vi "Actor Core.vi"(8 "error in":errorcluster, 11 "Nested in":refnum<class "UI.lvclass">) -> (0 "error out":errorcluster, 3 "Actor out":refnum<class "Actor.lvclass">)   [LabVIEW 2020, in "UI.lvlib" / "UI.lvclass"]
doc: "(<B>Filename</B>: Actor Framework.lvlib:Actor.lvclass:Actor Core.vi)\n\nReceives messages to the actor, reacts to them, and initiates any error handling that may shut the actor down.\n\nDescendant classes may override this VI to append parallel tasks for the actor to complete while it handles messages. Overrides use the Call Parent Method node."
uses:
  UI.lvclass
  C:/Program Files (x86)/National Instruments/LabVIEW 2020/vi.lib/ActorFramework/Actor/Actor.lvclass
  <vilib>/ActorFramework/Actor/Actor.lvclass
  Turnos/Turnos.lvclass
  Paquetes/Paquetes.lvclass
  Dinero/Dinero.lvclass
  Contabilidad/Contabilidad.lvclass
  UI.lvclass/UI.ctl
  Turnos/Turnos.lvclass/Turnos.ctl
  Paquetes/Paquetes.lvclass/Paquetes.ctl
  Dinero/Dinero.lvclass/Dinero.ctl
  <vilib>/ActorFramework/Actor/Actor.lvclass/Actor.ctl
  <vilib>/ActorFramework/Message Enqueuer/Message Enqueuer.lvclass/Message Enqueuer.ctl
  UI Messages/New Credit and cambio to Dinero Msg/New Credit and cambio to Dinero Msg.lvclass/New Credit and cambio to Dinero Msg.ctl
  UI Messages/Verificar Credito Msg/Verificar Credito Msg.lvclass/Verificar Credito Msg.ctl
  UI Messages/UI Mensaje to Paquetes Msg/UI Mensaje to Paquetes Msg.lvclass/UI Mensaje to Paquetes Msg.ctl
  UI Messages/Servicio to contabilidad Msg/Servicio to contabilidad Msg.lvclass/Servicio to contabilidad Msg.ctl
  <vilib>/ActorFramework/Message Enqueuer/Init from Existing Queue.vi
  <vilib>/ActorFramework/Message Enqueuer/Enqueue.vi
  <vilib>/ActorFramework/Stop Msg/Stop Msg.lvclass
  C:/Program Files (x86)/National Instruments/LabVIEW 2020/vi.lib/ActorFramework/Message/Message.lvclass
  UI Messages/New Credit and cambio to Dinero Msg/New Credit and cambio to Dinero Msg.lvclass
  UI Messages/Verificar Credito Msg/Verificar Credito Msg.lvclass
  UI Messages/UI Mensaje to Paquetes Msg/UI Mensaje to Paquetes Msg.lvclass
  UI Messages/Servicio to contabilidad Msg/Servicio to contabilidad Msg.lvclass
  <vilib>/ActorFramework/Message Priority Queue/Priority Enqueue.vi
  <vilib>/ActorFramework/Message Enqueuer/Message Enqueuer.lvclass
  UI Messages/Table to Turnos Msg/Table to Turnos Msg.lvclass
panel:
  out "New Credit":i32
  out "SERIVICIO":string
  out "Cambio":i32
  out "Credito":i32
  in  "Contabilidad":bool
  in  "Stop Total":bool
  in  "Stop":bool
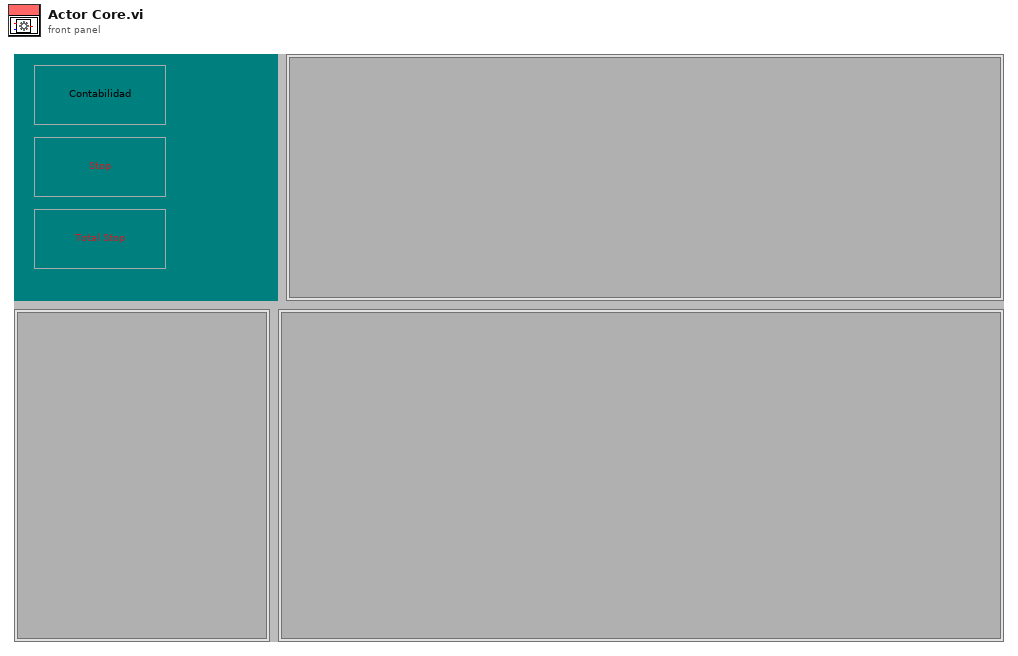
[diagram p1: front panel]
types:
  T1 = cluster{"Stop":refnum<user-event>, "Credito":refnum<user-event>, "Cambio":refnum<user-event>, "SERIVICIO":refnum<user-event>, "Mensaje":refnum<user-event>, "New Credit":refnum<user-event>, "Tabla estatus":refnum<user-event>}
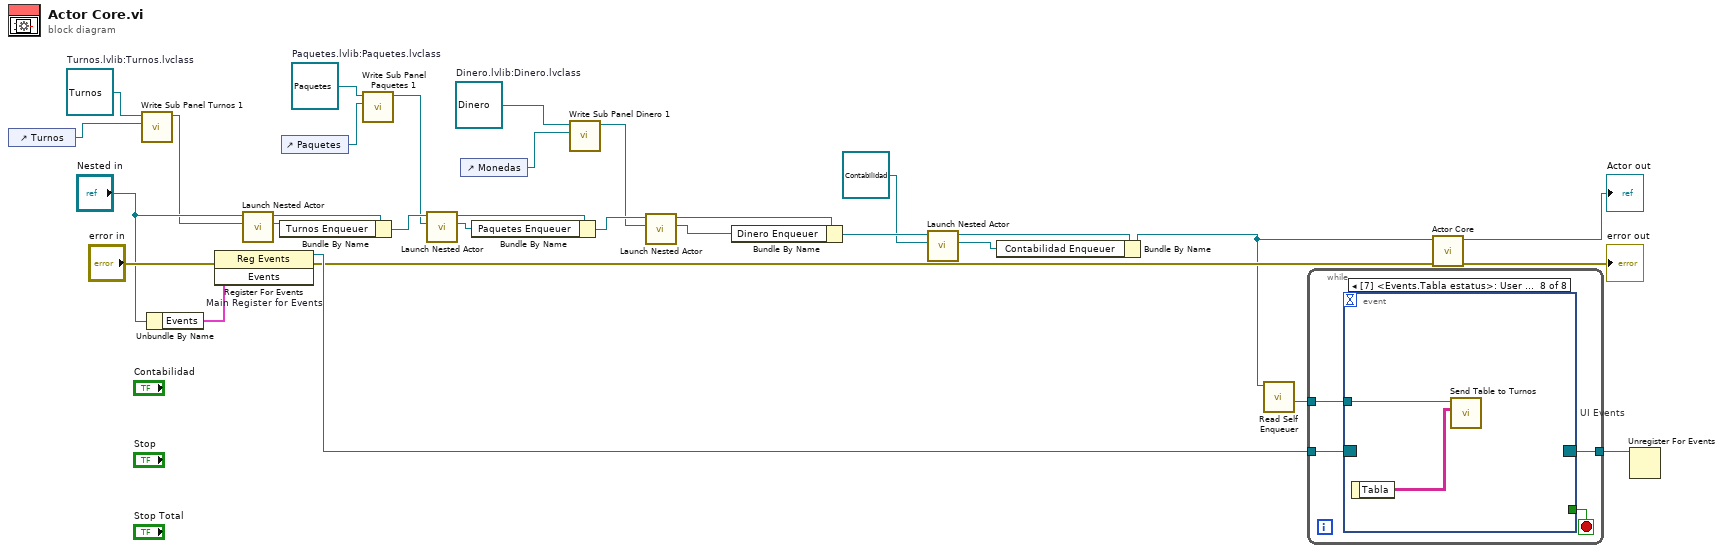
[diagram p0: block diagram]
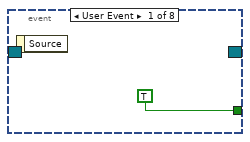
[diagram p2: hidden frame]
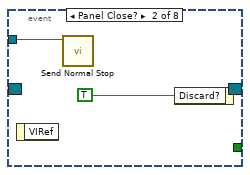
[diagram p3: hidden frame]
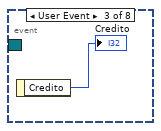
[diagram p4: hidden frame]
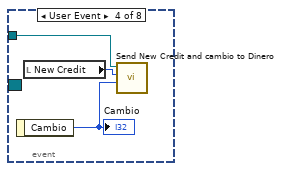
[diagram p5: hidden frame]
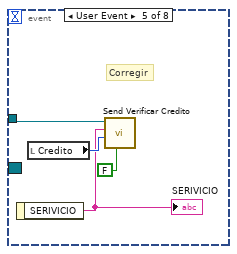
[diagram p6: hidden frame]
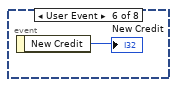
[diagram p7: hidden frame]
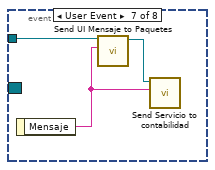
[diagram p8: hidden frame]
diagram:
  w10 = refnum<class "Dinero.lvclass"> refnum  # Dinero.lvlib:Dinero.lvclass
  w17 = refnum<class "Paquetes.lvclass"> refnum  # Paquetes.lvlib:Paquetes.lvclass
  w23 = refnum<class "Turnos.lvclass"> refnum  # Turnos.lvlib:Turnos.lvclass
  n1 = control-ref of="Turnos"() -> (w21:refnum<vi>)
  n2 = call "Write Sub Panel Turnos 1.vi"("Sub Panel Turnos"=w21, "Turnos in"=w23) -> ("Turnos out"=w20:refnum<class "Turnos.lvclass">)  [unwired: 8 in, 1 out]
  n3 = Unbundle By Name("Nested in") -> ("Events"=w28:T1)
  n4 = register-events "Main Register for Events"(error in="error in", w28) -> (reference out=w29:refnum<event-registration>, error out=w24:errorcluster)  [unwired: 1 in]
  n5 = call <vilib>:"Launch Nested Actor.vi"("Nested Actor"=w20, "Caller Actor in"="Nested in") -> ("Nested Actor's Enqueuer"=w18:refnum<class "Message Enqueuer.lvclass">, "Caller Actor out"=w19:refnum<class "UI.lvclass">)  [unwired: 7 in, 1 out]
  n6 = Bundle By Name(cluster=w19, "Turnos Enqueuer"=w18) -> (w15:refnum<class "UI.lvclass">)
  n7 = control-ref of="Paquetes"() -> (w16:refnum<vi>)
  n8 = call "Write Sub Panel Paquetes 1.vi"("Sub Panel Paquetes"=w16, "Paquetes in"=w17) -> ("Paquetes out"=w14:refnum<class "Paquetes.lvclass">)  [unwired: 8 in, 1 out]
  n9 = call <vilib>:"Launch Nested Actor.vi"("Nested Actor"=w14, "Caller Actor in"=w15) -> ("Nested Actor's Enqueuer"=w12:refnum<class "Message Enqueuer.lvclass">, "Caller Actor out"=w13:refnum<class "UI.lvclass">)  [unwired: 7 in, 1 out]
  n10 = control-ref of="Monedas"() -> (w9:refnum<vi>)
  n11 = Bundle By Name(cluster=w13, "Paquetes Enqueuer"=w12) -> (w11:refnum<class "UI.lvclass">)
  n12 = call "Write Sub Panel Dinero 1.vi"("Sub Panel Dinero"=w9, "Dinero in"=w10) -> ("Dinero out"=w8:refnum<class "Dinero.lvclass">)  [unwired: 8 in, 1 out]
  n13 = call <vilib>:"Launch Nested Actor.vi"("Nested Actor"=w8, "Caller Actor in"=w11) -> ("Nested Actor's Enqueuer"=w6:refnum<class "Message Enqueuer.lvclass">, "Caller Actor out"=w7:refnum<class "UI.lvclass">)  [unwired: 7 in, 1 out]
  n14 = Bundle By Name(cluster=w7, "Dinero Enqueuer"=w6) -> (w5:refnum<class "UI.lvclass">)
  n15 = call <vilib>:"Launch Nested Actor.vi"("Nested Actor"=refnum<class "Contabilidad.lvclass"> refnum ("Contabilidad.lvlib:Contabilidad.lvclass"), "Caller Actor in"=w5) -> ("Nested Actor's Enqueuer"=w2:refnum<class "Message Enqueuer.lvclass">, "Caller Actor out"=w4:refnum<class "UI.lvclass">)  [unwired: 7 in, 1 out]
  n16 = Bundle By Name(cluster=w4, "Contabilidad Enqueuer"=w2) -> (w3:refnum<class "UI.lvclass">)
  n17 = call <vilib>:"Read Self Enqueuer.vi"("Actor"=w3) -> ("Self Enqueuer"=w26:refnum<class "Message Enqueuer.lvclass">)  [unwired: 10 in]
  n18 = while {
    tunnel: w29 -> [w35]
    tunnel: [w33] -> w27
    tunnel: w26 -> [w32]
    stop <- w34 stop-if-true
    n19 = event "UI Events" shown="[7] <Events.Tabla estatus>: User Event" {
      selector: w35 -> [_ _ _ _ _ _ _ _]
      dyn-events: [_ _ _ _ _ _ _ _] -> w33
      timeout: _ -> [_ _ _ _ _ _ _ _]
      tunnel: [TRUE _ _ _ _ _ _ _] -> w34
      tunnel: w32 -> [_ w37 _ w41 w45 _ w50 w52]
      event User Event {
        n20 = event-data() -> ()  [unwired: 1 in, 1 out]
      }
      event Panel Close? {
        n21 = event-data() -> ()  [unwired: 1 in, 1 out]
        n22 = call <vilib>:"Send Normal Stop.vi"("Message Enqueuer"=w37) -> ()  [unwired: 10 in, 1 out]
        n23 = event-data("Discard?"=TRUE) -> ()  [unwired: 1 in, 1 out]
      }
      event User Event {
        n24 = event-data() -> ("Credito"=→"Credito":i32)  [unwired: 1 in]
      }
      event User Event {
        n25 = event-data() -> ("Cambio"=w42:i32)  [unwired: 1 in]
        "Cambio" <- w42
        n26 = local read "New Credit"() -> (w40:i32)
        n27 = call "Send New Credit and cambio to Dinero.vi"("Cambio"=w42, "Credito"=w40, "Message Enqueuer"=w41) -> ()  [unwired: 7 in, 2 out]
      }
      event User Event {
        # "Corregir"
        n28 = event-data() -> ("SERIVICIO"=w43:string)  [unwired: 1 in]
        "SERIVICIO" <- w43
        n29 = local read "Credito"() -> (w46:i32)
        n30 = call "Send Verificar Credito.vi"("STOP"=FALSE, "Credito"=w46, "Servicio"=w43, "Message Enqueuer"=w45) -> ()  [unwired: 6 in, 2 out]
      }
      event User Event {
        n31 = event-data() -> ("New Credit"=→"New Credit":i32)  [unwired: 1 in]
      }
      event User Event {
        n32 = event-data() -> ("Mensaje"=w48:string)  [unwired: 1 in]
        n33 = call "Send UI Mensaje to Paquetes.vi"("Mensaje"=w48, "Message Enqueuer"=w50) -> ("Message Enqueuer out"=w49:refnum<class "Message Enqueuer.lvclass">)  [unwired: 8 in, 1 out]
        n34 = call "Send Servicio to contabilidad.vi"("Servicio seleccionado"=w48, "Message Enqueuer"=w49) -> ()  [unwired: 8 in, 2 out]
      }
      event User Event {
        n35 = event-data() -> ("Tabla"=w51:string[][])  [unwired: 1 in]
        n36 = call "Send Table to Turnos.vi"("Tabla estatus"=w51, "Message Enqueuer"=w52) -> ()  [unwired: 8 in, 2 out]
      }
    }
  }
  n37 = call-parent "Actor Core.vi"("error in"=w24, "Actor in"=w3) -> ("error out"=→"error out":errorcluster, "Actor out"=→"Actor out":refnum<class "Actor.lvclass">)  [unwired: 8 in]
  n38 = Unregister For Events(event registration refnum=w27) -> ()  [unwired: 1 in, 1 out]
